vi "Avocent_Device_GUI.vi"() -> ()   [LabVIEW 2013]
doc: "Example of using standard HTTP protocol for recieving a web site (the HTML source)\n\n\nThis example uses the GET command. For general information about the HTTP protocol and other commands go to\nhttp://www.w3.org/Protocols\n\n\nBjornar Svingen\nbjornar.svingen@sintef.no bjornar.svingen@ktv.no"
uses:
  shared programs/GUI_Template/GUI_master/tcp_new_data_event.ctl
  shared programs/GUI_Template/GUI_master/tcp new data cluster.ctl
  <vilib>/Utility/config.llb/Read Key (String).vi
  <vilib>/Utility/config.llb/NI_LVConfig.lvlib
panel:
  in  "timeout::1":i32=6000 caption="timeout ms" min=0 max=0
  in  "turn selected OFF":bool
  in  "turn selected ON":bool
  out "Avocent Labels Av1":string[](array[string])
  in  "Set switches":bool[](array[boolean])=[FALSE, FALSE, FALSE, FALSE, FALSE, FALSE, FALSE, FALSE, FALSE, FALSE, FALSE, FALSE, FALSE, FALSE, FALSE, FALSE] caption="Set Switches"
  in  "Avocent IP::1":string caption="Avocent  IP"
  out "port: P::1":bool caption="port: P"
  out "port: O::1":bool caption="port: O"
  out "port: N::1":bool caption="port: N"
  out "port: M::1":bool caption="port: M"
  out "port: L::1":bool caption="port: L"
  out "port: K::1":bool caption="port: K"
  out "port: J::1":bool caption="port: J"
  out "port: I::1":bool caption="port: I"
  out "port: H::1":bool caption="port: H"
  out "port: G::1":bool caption="port: G"
  out "port: F::1":bool caption="port: F"
  out "port: E::1":bool caption="port: E"
  out "port: D::1":bool caption="port: D"
  out "port: C::1":bool caption="port: C"
  out "port: B::1":bool caption="port: B"
  out "port: A::1":bool caption="port: A"
  out "tcp data event 2":T1
  out "GUIdevice 1":string="Avocent-PSU-downstream"
  in  "Set to all on/off av1":bool
  in  "toggle av1":bool
  in  "Set to current values":bool
  out "Power indicator":bool[](array[boolean])=[FALSE, TRUE, TRUE, FALSE, TRUE, TRUE, TRUE, TRUE, TRUE, TRUE, TRUE, FALSE, TRUE, TRUE, TRUE, FALSE, FALSE, FALSE, FALSE, FALSE, FALSE, FALSE, FALSE, FALSE, FALSE, FALSE, FALSE, FALSE, FALSE, FALSE, FALSE, FALSE]
  in  "Get status":bool
  in  "send command":bool
  in  "Exit":bool
  out "Error":T2
  # "Power indicator"
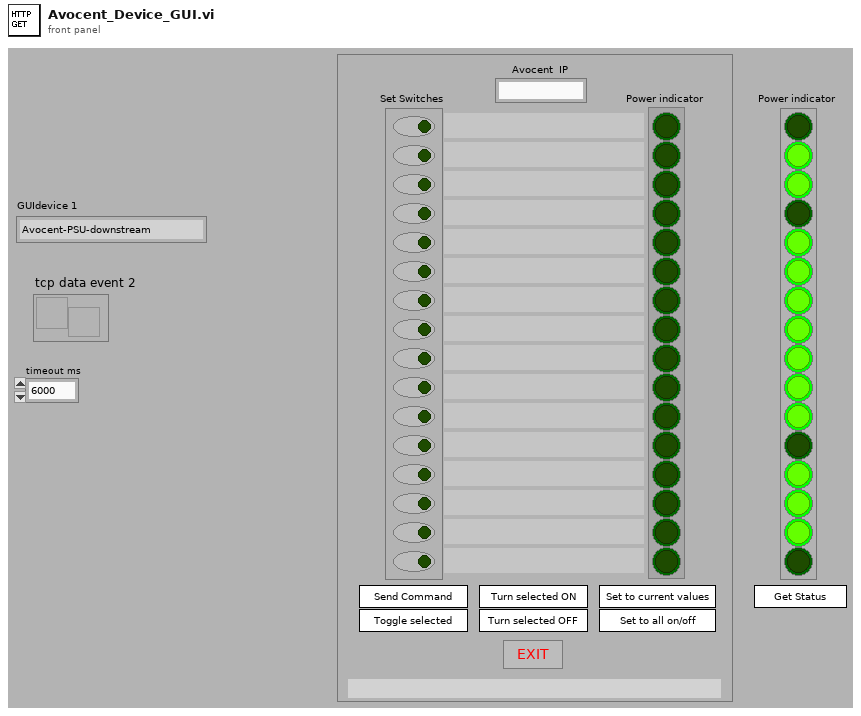
[diagram p1: front panel]
types:
  T1 = typedef "tcp_new_data_event.ctl" = refnum<user-event>
  T2 = cluster{"status":bool, "code":i32, "UDP error message":string}
  T3 = enum32{"invalid app kind", "Development System", "Run Time System", "Student Edition", "Embedded LabVIEW", "Evaluation", "Custom"}
  T4 = typedef "tcp new data cluster.ctl" = cluster{"EventEnum":enum16{"new data", "connection status update"}, "Device name":string}
  T5 = enum32{"Invalid", "Standard", "Closed", "Hidden", "Minimized", "Maximized"}
  T6 = cluster{"Core":cluster{"Current VI Reference":refnum<vi>, "Close Panel on Exit?":bool}, "HTTP Command":string, "Set Switch Status":bool[], "Power Status":string, "Toggle On/Off":bool, "Set all On/Off":bool, "SuperGUI":cluster{"STOP queue":refnum<queue>, "SuperGUI ref":refnum<vi>, "event reg":refnum<event-registration>}, "Stage Device list":string[], "Avocent IP":string}
  T7 = cluster{"STOP queue":refnum<queue>, "SuperGUI ref":refnum<vi>, "event reg":refnum<event-registration>}
  T8 = cluster{"Current VI Reference":refnum<vi>, "Close Panel on Exit?":bool}
  T9 = typedef "NI_LVConfig.lvlib/Config Data RefNum.ctl" = refnum<k1>
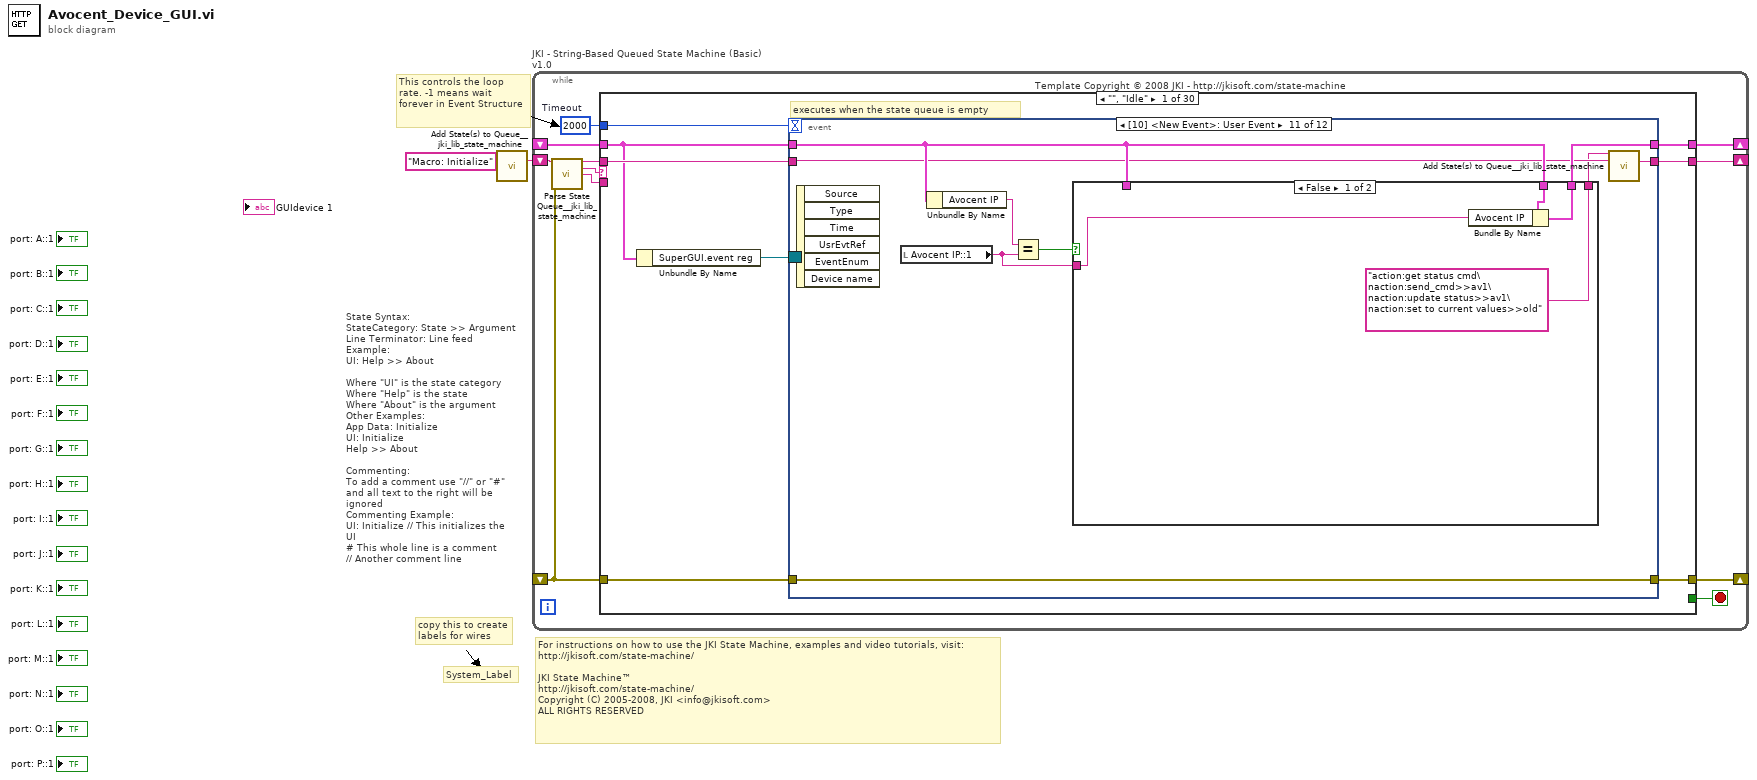
[diagram p0: block diagram]
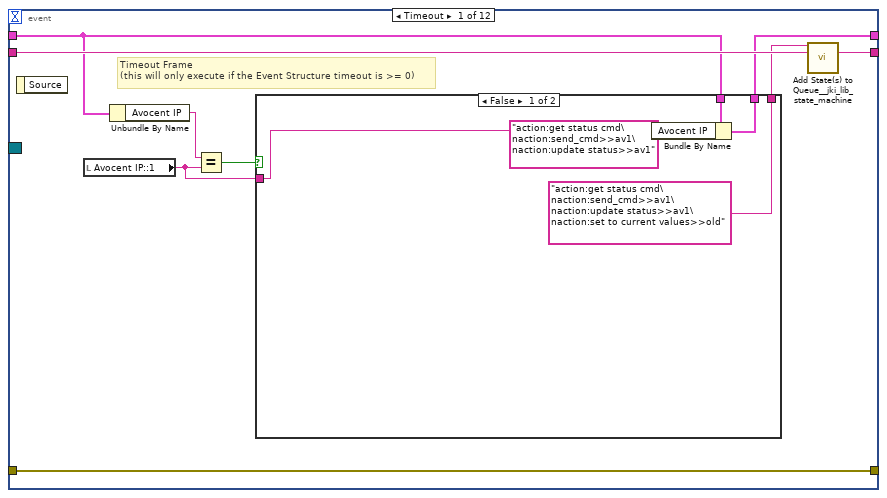
[diagram p2: hidden frame]
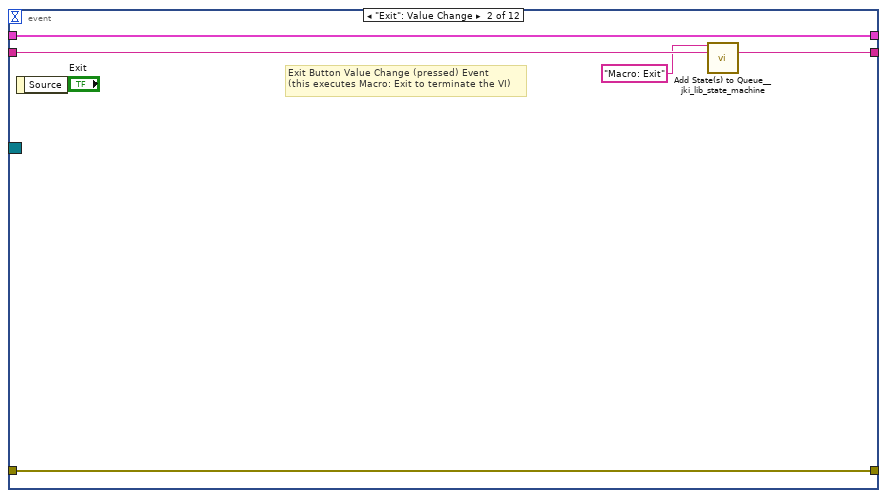
[diagram p4: hidden frame]
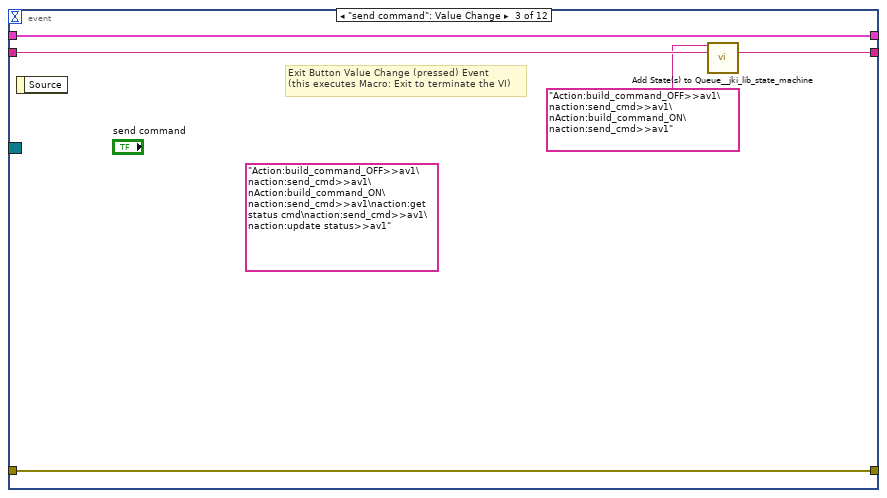
[diagram p5: hidden frame]
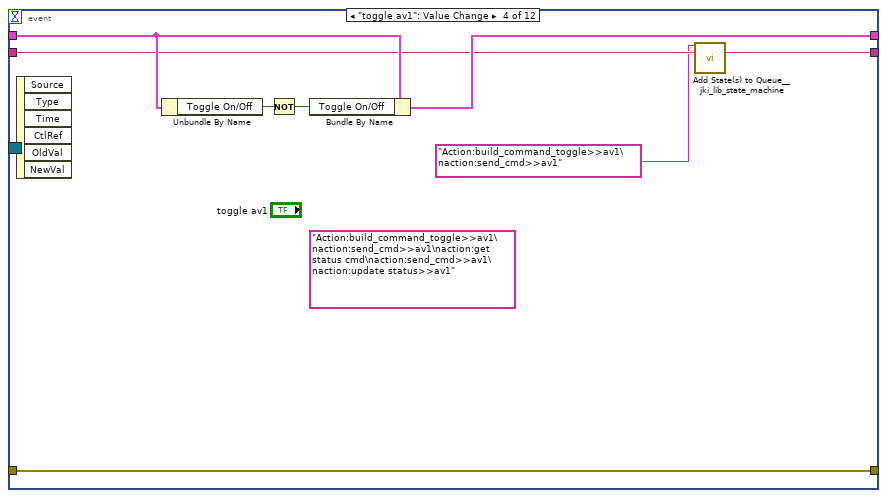
[diagram p6: hidden frame]
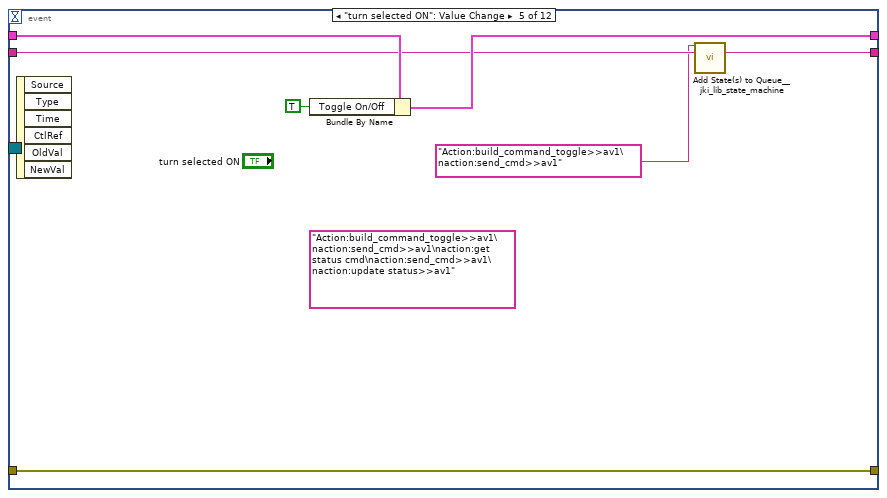
[diagram p7: hidden frame]
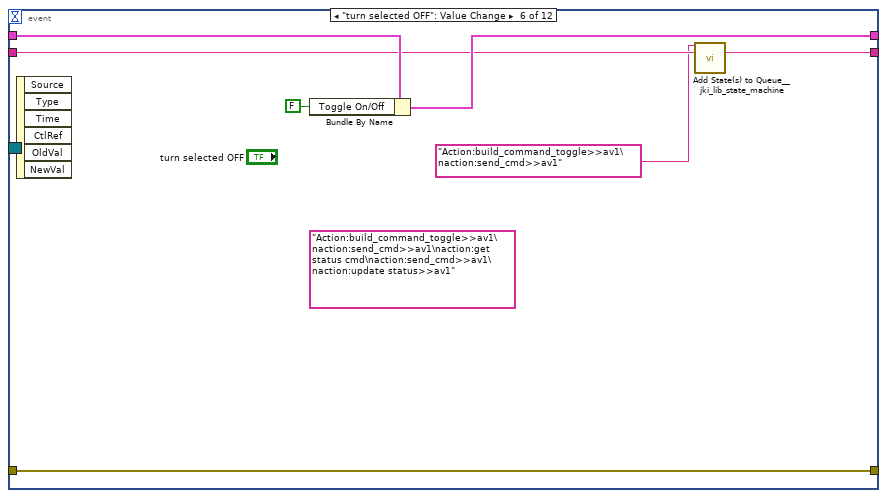
[diagram p8: hidden frame]
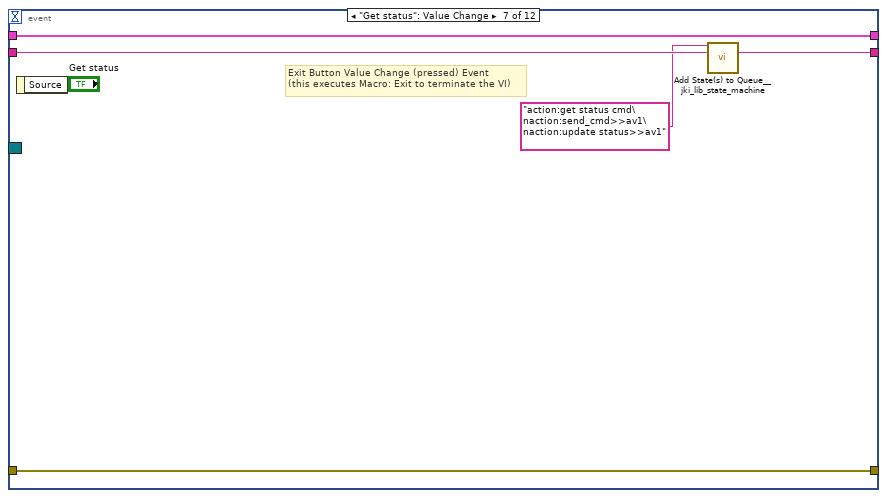
[diagram p9: hidden frame]
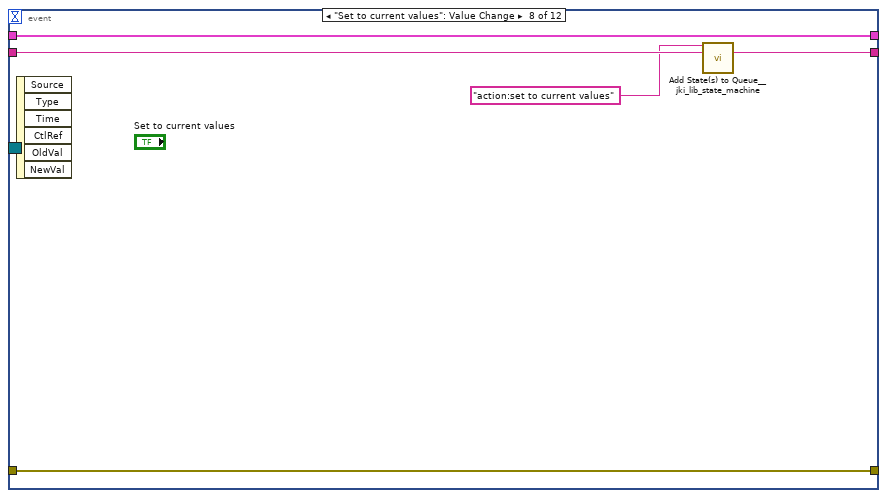
[diagram p10: hidden frame]
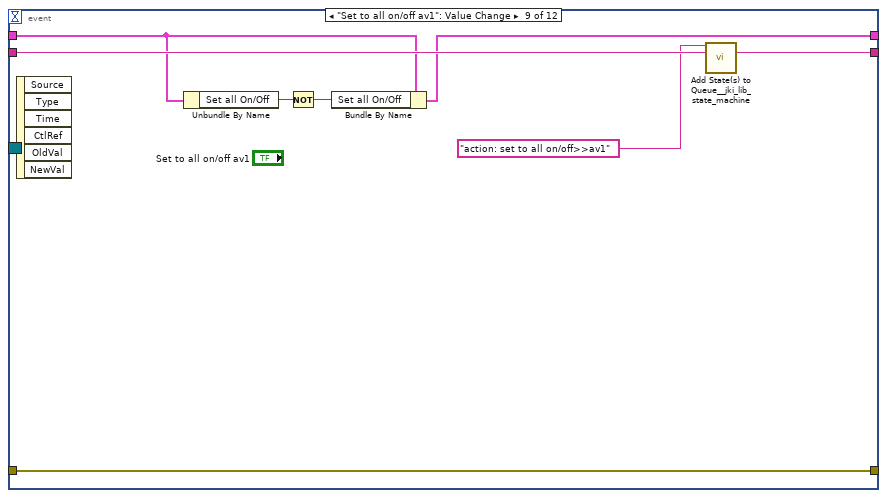
[diagram p11: hidden frame]
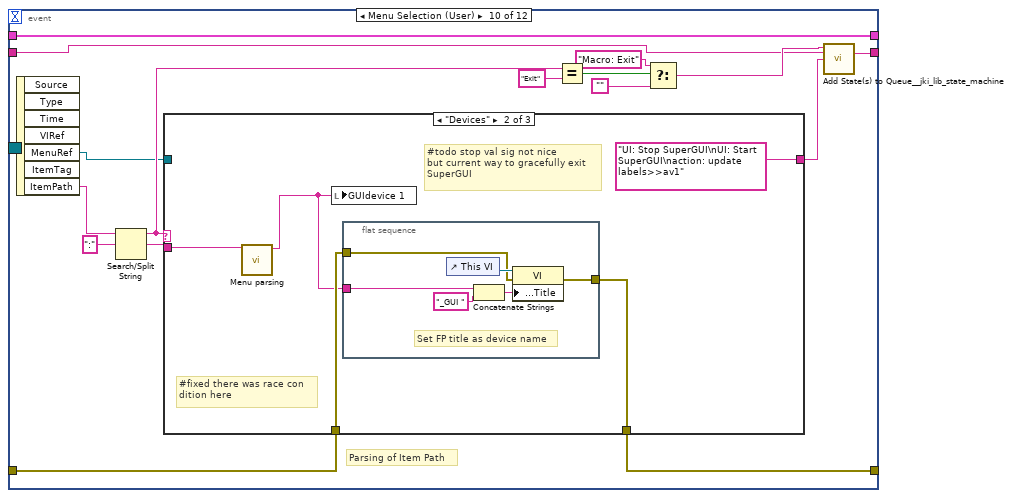
[diagram p12: hidden frame]
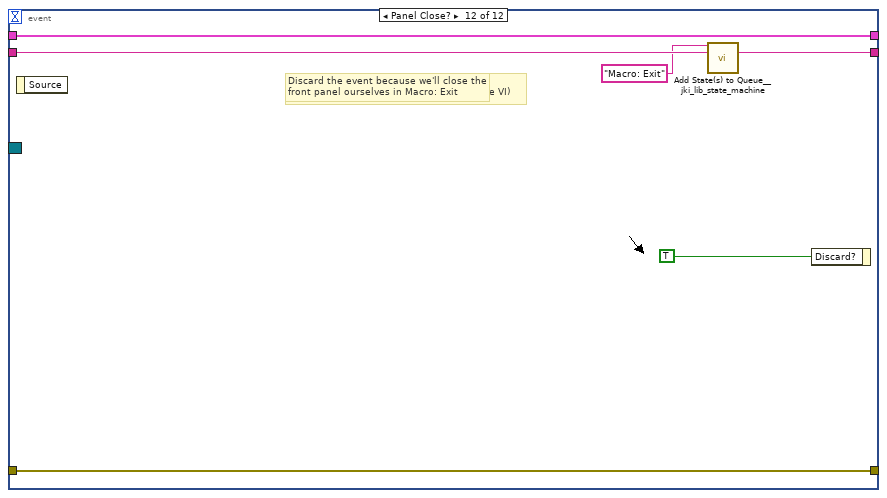
[diagram p16: hidden frame]
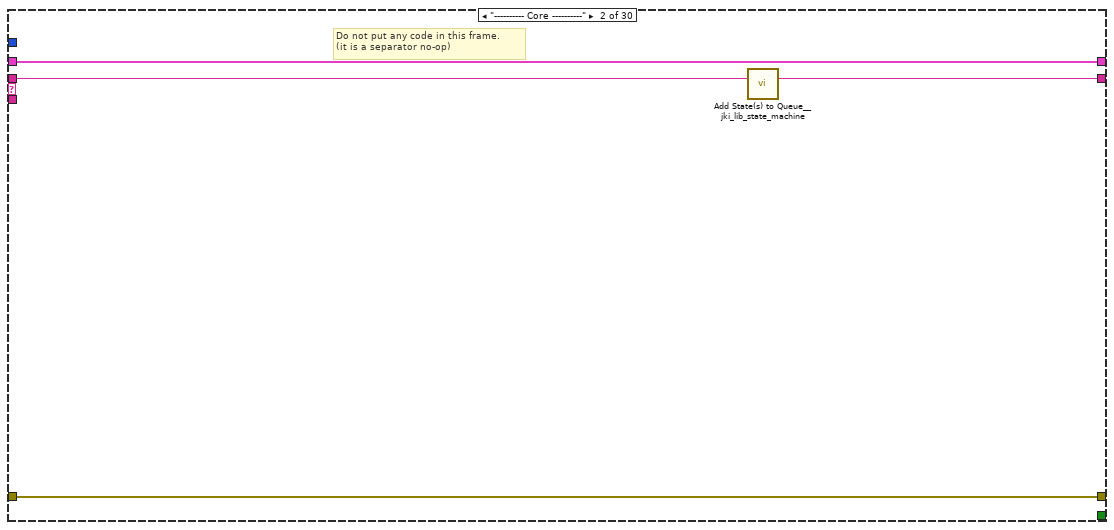
[diagram p17: hidden frame]
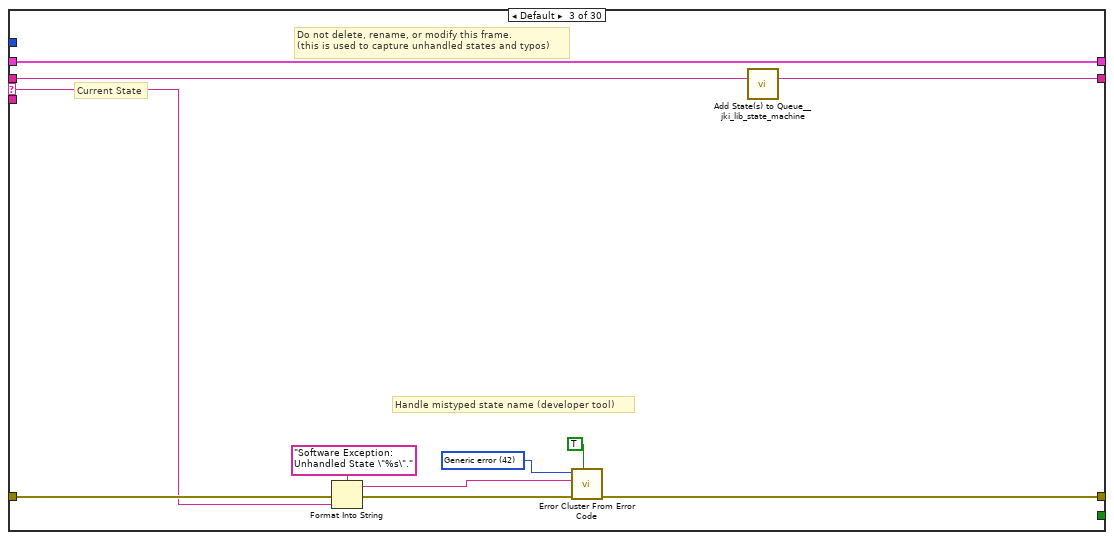
[diagram p18: hidden frame]
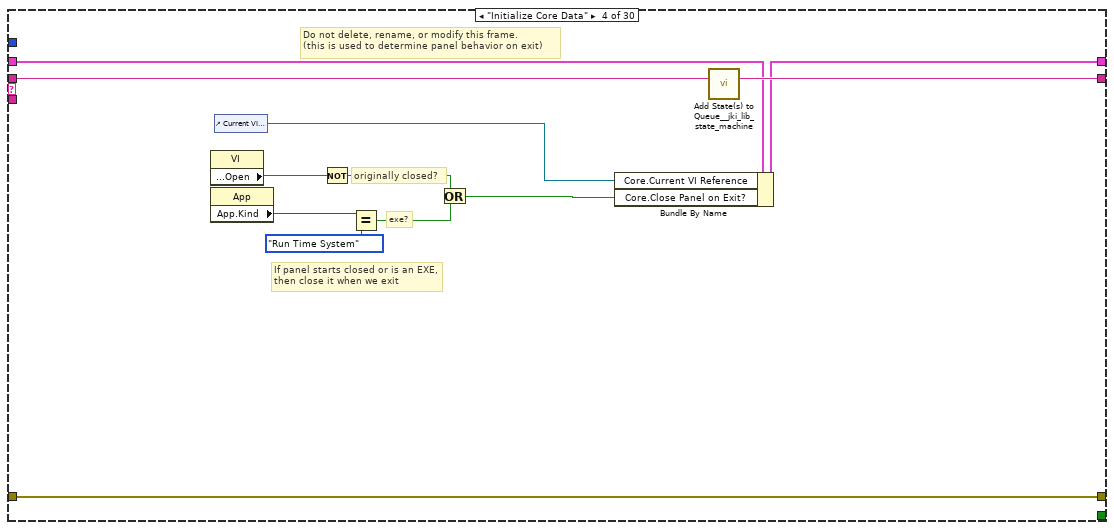
[diagram p19: hidden frame]
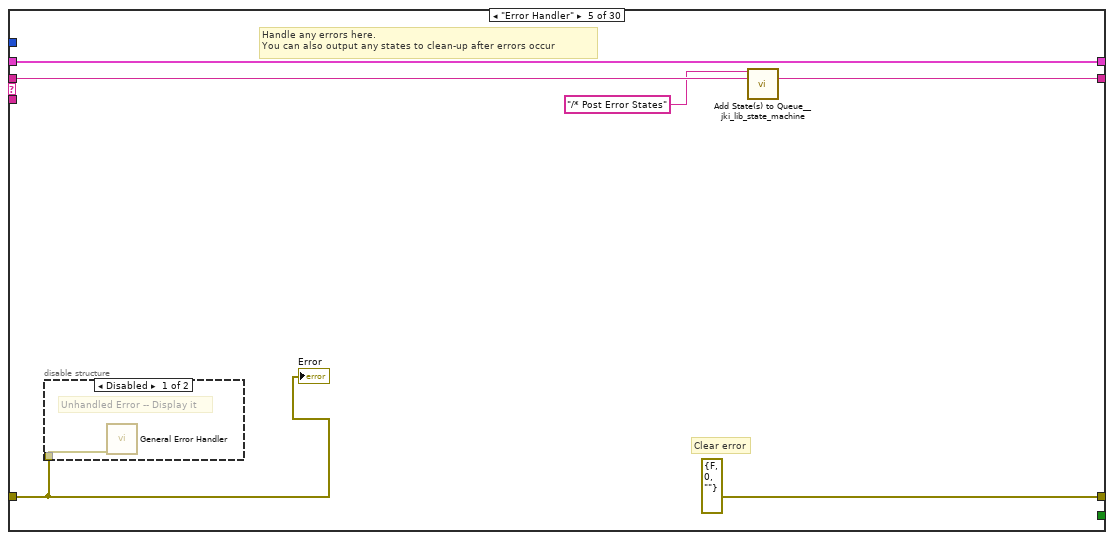
[diagram p20: hidden frame]
diagram:
  # "For instructions on how to use the JKI State Machine, examples and video tutorials, visit:\nhttp://jkisoft.com/state-machine/\n\nJKI State Machine™\nhttp://jkisoft.com/state-machine/\nCopyright (C) 2005-2008, JKI <info@jkisoft.com>\nALL RIGHTS RESERVED"
  # "State Syntax:\nStateCategory: State >> Argument\nLine Terminator: Line feed\nExample:\nUI: Help >> About\n\nWhere \"UI\" is the state category\nWhere \"Help\" is the state\nWhere \"About\" is the argument\nOther Examples:\nApp Data: Initialize\nUI: Initialize\nHelp >> About\n\nCommenting:\nTo add a comment use \"//\" or \"#\" and all text to the right will be ignored\nCommenting Example:\nUI: Initialize // This initializes the UI\n# This whole line is a comment\n// Another comment line"
  # "copy this to create labels for wires"
  # "This controls the loop rate. -1 means wait forever in Event Structure"
  # "System_Label"
  n1 = call <vilib>:"Add State(s) to Queue__jki_lib_state_machine.vi"("State(s) in (\"\")"="Macro: Initialize") -> ("States Out"=w2:string)  [unwired: 14 in]
  n2 = while "JKI - String-Based Queued State Machine (Basic) v1.0" {
    shift-right: [w6] -> _
    shift-left: _ -> [w5]
    shift-right: [w9] -> _
    shift-left: _ -> [w3]
    shift-right: [w8] -> _
    shift-left: w2 -> [w10]
    stop <- w7 stop-if-true
    w4 = 2000  # Timeout
    # "Template Copyright © 2008 JKI - http://jkisoft.com/state-machine"
    n3 = call <vilib>:"Parse State Queue__jki_lib_state_machine.vi"("State Queue"=w10, "Error In (no error)"=w3) -> ("Remaining States"=w12:string, "Current State"=w13:string, "Arguments"=w11:string)  [unwired: 11 in]
    n4 = case shown="\"\", \"Idle\"" w13 {
      selector: w13 -> [_ _ w139 _ _ _ _ _ _ _ _ _ _ _ _ _ _ _ _ _ _ _ _ _ _ _ _ _ _ _]
      tunnel: w12 -> [w21 w138 w143 w161 w167 w173 w177 w190 w196 w200 w208 w210 w231 w270 w282 w295 w306 w332 w337 w347 w351 w354 w375 w392 w397 w413 w429 w435 w463 w488]
      tunnel: w11 -> [_ _ _ _ _ _ _ _ _ _ _ _ _ _ _ w290 w300 _ _ _ _ w357 w376 _ w399 w416 _ w430 w464 w477]
      tunnel: w5 -> [w15 w135 w141 w152 w164 w171 w174 _ w191 w197 w206 w209 w232 w267 w286 w293 w302 w329 w334 w344 w348 w359 w379 w388 w398 w417 w426 w433 w459 w489]
      tunnel: [w19 w136 w145 w158 errorcluster {"status"=FALSE, "code"=0, "source"=""} ("error out") w170 w175 w187 w192 w198 w204 w212 w233 w266 w284 w291 w303 w330 w335 w345 w349 w362 w373 w390 w400 w414 w427 w431 w465 w480] -> w9
      tunnel: w3 -> [w18 w136 w144 w158 w162 w170 w175 w187 w193 w198 w205 w213 w234 w265 w285 w292 w304 w330 w335 w345 w349 w356 w374 w390 w401 w415 w427 w432 w466 w476]
      tunnel: [w20 w137 w142 w160 w166 w172 w176 w189 w195 w199 w207 w211 w231 w269 w283 w294 w305 w331 w336 w346 w350 w364 w380 w391 w403 w418 w428 w434 w467 w488] -> w8
      tunnel: [_ _ _ _ _ TRUE _ _ _ _ _ _ _ _ _ _ _ _ _ _ _ _ _ _ _ _ _ _ _ _] -> w7
      tunnel: [w17 w135 w141 w159 w164 w171 w174 w188 w191 w197 w206 w209 w232 w268 w286 w293 w302 w329 w334 w344 w348 w358 w377 w389 w402 w417 w425 w433 w459 w489] -> w6
      tunnel: w4 -> [w16 _ _ _ _ _ _ _ _ _ _ _ _ _ _ _ _ _ _ _ _ _ _ _ _ _ _ _ _ _]
      frame "", "Idle" {
        # "executes when the state queue is empty"
        n5 = Unbundle By Name(w15) -> ("SuperGUI.event reg"=w14:refnum<event-registration>)
        n6 = event shown="[10] <New Event>: User Event" {
          selector: w14 -> [_ _ _ _ _ _ _ _ _ _ _ _]
          dyn-events: _ -> [_ _ _ _ _ _ _ _ _ _ _ _]
          timeout: w16 -> [_ _ _ _ _ _ _ _ _ _ _ _]
          tunnel: w21 -> [w30 w40 w45 w48 w57 w64 w72 w74 w83 w89 w116 w134]
          tunnel: [w29 w39 w44 w47 w56 w63 w71 w75 w84 w87 w117 w133] -> w20
          tunnel: w15 -> [w23 w37 w42 w51 w58 w65 w69 w77 w79 w88 w119 w131]
          tunnel: [w28 w38 w43 w53 w60 w67 w70 w76 w85 w93 w123 w132] -> w19
          tunnel: w18 -> [w28 w38 w43 w53 w60 w67 w70 w76 w85 w92 w123 w132]
          tunnel: [w22 w37 w42 w52 w59 w66 w69 w77 w78 w88 w121 w131] -> w17
          event Timeout {
            (unwired) "action:get status cmd\naction:send_cmd>>av1\naction:update status>>av1"
            # "Timeout Frame\n(this will only execute if the Event Structure timeout is >= 0)"
            n7 = event-data() -> ()  [unwired: 1 in, 1 out]
            n8 = local read "Avocent IP::1"() -> (w25:string)
            n9 = Unbundle By Name(w23) -> ("Avocent IP"=w27:string)
            n10 = Equal?(x=w27, y=w25) -> (x = y?=w26:bool)
            n11 = case shown="False" w26 {
              tunnel: w23 -> [w34 w35]
              tunnel: [w33 w35] -> w22
              tunnel: w25 -> [w32 _]
              tunnel: ["action:get status cmd\naction:send_cmd>>av1\naction:update status>>av1\naction:set to current values>>old" ("State(s) in Front (\"\")") _] -> w24
              frame False {
                n12 = Bundle By Name(cluster=w34, "Avocent IP"=w32) -> (w33:T6)
              }
              frame True {
              }
            }
            n13 = call <vilib>:"Add State(s) to Queue__jki_lib_state_machine.vi"("State(s) in Front (\"\")"=w24, "State(s) in (\"\")"=w30) -> ("States Out"=w29:string)  [unwired: 13 in]
          }
          event "Exit": Value Change {
            # "Exit Button Value Change (pressed) Event\n(this executes Macro: Exit to terminate the VI)"
            n14 = event-data() -> ()  [unwired: 1 in, 1 out]
            n15 = call <vilib>:"Add State(s) to Queue__jki_lib_state_machine.vi"("State(s) in Front (\"\")"="Macro: Exit", "State(s) in (\"\")"=w40) -> ("States Out"=w39:string)  [unwired: 13 in]
          }
          event "send command": Value Change {
            (unwired) "Action:build_command_OFF>>av1\naction:send_cmd>>av1\nAction:build_command_ON\naction:send_cmd>>av1\naction:get status cmd\naction:send_cmd>>av1\naction:update status>>av1"
            # "Exit Button Value Change (pressed) Event\n(this executes Macro: Exit to terminate the VI)"
            n16 = event-data() -> ()  [unwired: 1 in, 1 out]
            n17 = call <vilib>:"Add State(s) to Queue__jki_lib_state_machine.vi"("State(s) in Front (\"\")"="Action:build_command_OFF>>av1\naction:send_cmd>>av1\nAction:build_command_ON\naction:send_cmd>>av1", "State(s) in (\"\")"=w45) -> ("States Out"=w44:string)  [unwired: 13 in]
          }
          event "toggle av1": Value Change {
            (unwired) "Action:build_command_toggle>>av1\naction:send_cmd>>av1\naction:get status cmd\naction:send_cmd>>av1\naction:update status>>av1"
            n18 = event-data() -> ()  [unwired: 1 in, 6 out]
            n19 = Unbundle By Name(w51) -> ("Toggle On/Off"=w50:bool)
            n20 = Not(x=w50) -> (.not. x?=w49:bool)
            n21 = Bundle By Name(cluster=w51, "Toggle On/Off"=w49) -> (w52:T6)
            n22 = call <vilib>:"Add State(s) to Queue__jki_lib_state_machine.vi"("State(s) in Front (\"\")"="Action:build_command_toggle>>av1\naction:send_cmd>>av1", "State(s) in (\"\")"=w48) -> ("States Out"=w47:string)  [unwired: 13 in]
          }
          event "turn selected ON": Value Change {
            (unwired) "Action:build_command_toggle>>av1\naction:send_cmd>>av1\naction:get status cmd\naction:send_cmd>>av1\naction:update status>>av1"
            n23 = event-data() -> ()  [unwired: 1 in, 6 out]
            n24 = Bundle By Name(cluster=w58, "Toggle On/Off"=TRUE) -> (w59:T6)
            n25 = call <vilib>:"Add State(s) to Queue__jki_lib_state_machine.vi"("State(s) in Front (\"\")"="Action:build_command_toggle>>av1\naction:send_cmd>>av1", "State(s) in (\"\")"=w57) -> ("States Out"=w56:string)  [unwired: 13 in]
          }
          event "turn selected OFF": Value Change {
            (unwired) "Action:build_command_toggle>>av1\naction:send_cmd>>av1\naction:get status cmd\naction:send_cmd>>av1\naction:update status>>av1"
            n26 = event-data() -> ()  [unwired: 1 in, 6 out]
            n27 = Bundle By Name(cluster=w65, "Toggle On/Off"=FALSE) -> (w66:T6)
            n28 = call <vilib>:"Add State(s) to Queue__jki_lib_state_machine.vi"("State(s) in Front (\"\")"="Action:build_command_toggle>>av1\naction:send_cmd>>av1", "State(s) in (\"\")"=w64) -> ("States Out"=w63:string)  [unwired: 13 in]
          }
          event "Get status": Value Change {
            # "Exit Button Value Change (pressed) Event\n(this executes Macro: Exit to terminate the VI)"
            n29 = event-data() -> ()  [unwired: 1 in, 1 out]
            n30 = call <vilib>:"Add State(s) to Queue__jki_lib_state_machine.vi"("State(s) in Front (\"\")"="action:get status cmd\naction:send_cmd>>av1\naction:update status>>av1", "State(s) in (\"\")"=w72) -> ("States Out"=w71:string)  [unwired: 13 in]
          }
          event "Set to current values": Value Change {
            n31 = event-data() -> ()  [unwired: 1 in, 6 out]
            n32 = call <vilib>:"Add State(s) to Queue__jki_lib_state_machine.vi"("State(s) in Front (\"\")"="action:set to current values" ("State(s) in Front (\"\")"), "State(s) in (\"\")"=w74) -> ("States Out"=w75:string)  [unwired: 13 in]
          }
          event "Set to all on/off av1": Value Change {
            n33 = event-data() -> ()  [unwired: 1 in, 6 out]
            n34 = Unbundle By Name(w79) -> ("Set all On/Off"=w81:bool)
            n35 = Not(x=w81) -> (.not. x?=w80:bool)
            n36 = Bundle By Name(cluster=w79, "Set all On/Off"=w80) -> (w78:T6)
            n37 = call <vilib>:"Add State(s) to Queue__jki_lib_state_machine.vi"("State(s) in Front (\"\")"="action: set to all on/off>>av1" ("State(s) in Front (\"\")"), "State(s) in (\"\")"=w83) -> ("States Out"=w84:string)  [unwired: 13 in]
          }
          event Menu Selection (User) {
            # "Parsing of Item Path"
            n38 = event-data() -> ("MenuRef"=w91:refnum<k9>, "ItemPath"=w90:string)  [unwired: 1 in, 5 out]
            n39 = Search/Split String(string=w90, search string/char (-)=":") -> (substring before match=w100:string, match + rest of string=w94:string)  [unwired: 1 in, 1 out]
            n40 = case shown="\"Devices\"" w100 {
              tunnel: w94 -> [_ w107 _]
              tunnel: w91 -> [_ _ _]
              tunnel: w92 -> [w102 w106 w114]
              tunnel: [w102 w105 w114] -> w93
              tunnel: [_ "UI: Stop SuperGUI\nUI: Start SuperGUI\naction: update labels>>av1" _] -> w101
              frame "", Default {
              }
              frame "Devices" {
                # "#fixed there was race con\ndition here"
                # "#todo stop val sig not nice\nbut current way to gracefully exit\nSuperGUI"
                n41 = call "Menu parsing.vi"("ItemPath 3"=w107) -> ("ItemPath 2"=w103:string)  [unwired: 9 in, 1 out]
                n42 = local write "GUIdevice 1"(w103) -> ()
                n43 = flat-sequence {
                  tunnel: [w110] -> w105
                  tunnel: w106 -> [w109]
                  tunnel: w103 -> [w108]
                  frame #0 {
                    # "Set FP title as device name"
                    n44 = control-ref of="This VI"() -> (w113:refnum<vi>)
                    n45 = Concatenate Strings(w108, "_GUI ") -> (w112:string)
                    n46 = property class="VI"(reference=w113, error in=w109, "Front Panel.Title"=w112) -> (error out=w110:errorcluster)  [unwired: 1 out]
                  }
                }
              }
              frame "Exit" {
              }
            }
            n47 = Equal?(x=w100, y="Exit") -> (x = y?=w96:bool)
            n48 = Select(t="Macro: Exit", s=w96, f="") -> (s? t:f=w99:string)
            n49 = call <vilib>:"Add State(s) to Queue__jki_lib_state_machine.vi"("State(s) in Front (\"\")"=w99, "State(s) in (\"\")"=w89, "State(s) at Back (\"\")"=w101) -> ("States Out"=w87:string)  [unwired: 12 in]
          }
          event User Event {
            n50 = event-data() -> ()  [unwired: 1 in, 6 out]
            n51 = local read "Avocent IP::1"() -> (w118:string)
            n52 = Unbundle By Name(w119) -> ("Avocent IP"=w122:string)
            n53 = Equal?(x=w122, y=w118) -> (x = y?=w120:bool)
            n54 = case shown="False" w120 {
              tunnel: w119 -> [w127 w128]
              tunnel: [w126 w128] -> w121
              tunnel: w118 -> [w125 _]
              tunnel: w119 -> [_ _]
              tunnel: ["action:get status cmd\naction:send_cmd>>av1\naction:update status>>av1\naction:set to current values>>old" ("State(s) in Front (\"\")") _] -> w115
              frame False {
                n55 = Bundle By Name(cluster=w127, "Avocent IP"=w125) -> (w126:T6)
              }
              frame True {
              }
            }
            n56 = call <vilib>:"Add State(s) to Queue__jki_lib_state_machine.vi"("State(s) in Front (\"\")"=w115, "State(s) in (\"\")"=w116) -> ("States Out"=w117:string)  [unwired: 13 in]
          }
          event Panel Close? {
            # "Discard the event because we'll close the front panel ourselves in Macro: Exit"
            # "Close Panel button (pressed) Event\n(this executes Macro: Exit to terminate the VI)"
            n57 = event-data() -> ()  [unwired: 1 in, 1 out]
            n58 = call <vilib>:"Add State(s) to Queue__jki_lib_state_machine.vi"("State(s) in Front (\"\")"="Macro: Exit", "State(s) in (\"\")"=w134) -> ("States Out"=w133:string)  [unwired: 13 in]
            n59 = event-data("Discard?"=TRUE) -> ()  [unwired: 1 in, 1 out]
          }
        }
      }
      frame "---------- Core ----------" {
        # "Do not put any code in this frame.\n(it is a separator no-op)"
        n60 = call <vilib>:"Add State(s) to Queue__jki_lib_state_machine.vi"("State(s) in (\"\")"=w138) -> ("States Out"=w137:string)  [unwired: 14 in]
      }
      frame Default {
        w148 = 42 items=["No error", "Argument error", "Memory is full", "Out of zone", "End of file", "File already open", "Generic file I/O error", "File not found", "File permission error", "Disk is full", "Duplicate path", "Too many files open", "System feature not enabled", "Resource file not found", "Cannot add resource", "Resource not found", "Image not found", "Image memory error", "Pen does not exist", "Config type invalid", "Config token not found", "Config parse error", "Config memory error", "Bad external code format", "Bad external code offset", "External code not present", "Null window", "Destroy window error", "Null menu", "Print aborted", "Bad print record", "Print driver error", "Windows error during printing", "Memory error during printing", "Print dialog error", "Generic print error", "Invalid device refnum", "Device not found", "Device parameter error", "Device unit error", "Cannot open device", "Device call aborted", "Generic error", "Cancelled by user", "Object ID too low", "Object ID too high", "Object not in heap", "Unknown heap", "Unknown object (invalid DefProc)", "Unknown object (DefProc not in table)", "Message out of range", "Invalid (null) method", "Unknown message", "Manager call not supported", "Bad address", "Network operation in progress", "Network operation timed out", "Connection is busy", "Network attribute not supported", "Network error", "Address in use", "System out of memory", "Connection aborted", "Connection refused", "Not connected", "Already connected", "Connection closed", "Initialization error (interapplication manager)", "Bad occurrence", "Wait on unbound occurrence handler", "Occurrence queue overflow", "Datalog type conflict", "Unused", "Unrecognized type (interapplication manager)", "Memory corrupt", "Failed to make temporary DLL", "Old CIN version", "Drag socket not found", "Failed to load drop-object", "Failed to register OLE object", "Failed to release OLE object", "Format specifier type mismatch", "Unknown format specifier", "Too few format specifiers", "Too many format specifiers", "Scan failed", "Newer CIN version", "Error converting to variant", "Runtime menu error", "Password tampered", "Variant attribute not found", "Incompatible variant data type", "Event data is not available", "Event Store is not present", "Occurrence is not found", "Event Queue is not created", "Event info is not available", "Refnum passed is NULL", "Error retrieving Class GUID", "Error retrieving CoClass GUID", "Error retrieving TypeLib GUID.", "Bad built application magic bytes.", "Specific driver is different from the specific driver associated with the Logical Name.", "There is no session opened to the class driver.", "Max Error", "MAX - Error with config objects", "MAX - Error loading configuration", "MAX - Group not supported"]
        # "Current State"
        # "Do not delete, rename, or modify this frame.\n(this is used to capture unhandled states and typos)"
        # "Handle mistyped state name (developer tool)"
        n61 = Format Into String(format string="Software Exception: Unhandled State \"%s\"." ("message"), error in=w144, w139) -> (resulting string=w147:string, error out=w146:errorcluster)  [unwired: 1 in]
        n62 = call <vilib>:"Error Cluster From Error Code.vi"("show call chain? (False)"=TRUE, "error in (no error)"=w146, "error message (\"\")"=w147, "error code (0)"=w148) -> ("error out"=w145:errorcluster)  [unwired: 5 in]
        n63 = call <vilib>:"Add State(s) to Queue__jki_lib_state_machine.vi"("State(s) in (\"\")"=w143) -> ("States Out"=w142:string)  [unwired: 14 in]
      }
      frame "Initialize Core Data" {
        # "Do not delete, rename, or modify this frame.\n(this is used to determine panel behavior on exit)"
        # "originally closed?"
        # "exe?"
        # "If panel starts closed or is an EXE, then close it when we exit"
        n64 = property class="VI"() -> ("Front Panel.Open"=w157:bool)  [unwired: 2 in, 2 out]
        n65 = property class="App"() -> ("App.Kind"=w156:T3)  [unwired: 2 in, 2 out]
        n66 = control-ref of="Current VI Reference"() -> (w150:refnum<vi>)
        n67 = Not(x=w157) -> (.not. x?=w154:bool)
        n68 = Equal?(x=w156, y=T3."Run Time System" ("Application:Kind")) -> (x = y?=w153:bool)
        n69 = Or(x=w154, y=w153) -> (x .or. y?=w151:bool)
        n70 = Bundle By Name(cluster=w152, "Core.Current VI Reference"=w150, "Core.Close Panel on Exit?"=w151) -> (w159:T6)
        n71 = call <vilib>:"Add State(s) to Queue__jki_lib_state_machine.vi"("State(s) in (\"\")"=w161) -> ("States Out"=w160:string)  [unwired: 14 in]
      }
      frame "Error Handler" {
        # "Handle any errors here.\nYou can also output any states to clean-up after errors occur"
        # "Clear error"
        n72 = disable-structure shown="Disabled" {
          disable-tunnel: w162 -> [w168 _]
          frame Disabled {
            # "Unhandled Error -- Display it"
            n73 = call <vilib>:"General Error Handler.vi"("error in (no error)"=w168) -> ()  [unwired: 10 in, 5 out]
          }
          frame Enabled {
          }
        }
        n74 = call <vilib>:"Add State(s) to Queue__jki_lib_state_machine.vi"("State(s) in Front (\"\")"="/* Post Error States", "State(s) in (\"\")"=w167) -> ("States Out"=w166:string)  [unwired: 13 in]
        "Error" <- w162
      }
      frame "Exit" {
        # "Do not put any code in this frame.\n(No errors that occur here will be handled.)"
        n75 = call <vilib>:"Add State(s) to Queue__jki_lib_state_machine.vi"("State(s) in (\"\")"=w173) -> ("States Out"=w172:string)  [unwired: 14 in]
      }
      frame "---------- Data ----------" {
        # "Do not put any code in this frame.\n(It is a separator no-op. You can make a copy of this frame to create a new Data frame)"
        n76 = call <vilib>:"Add State(s) to Queue__jki_lib_state_machine.vi"("State(s) in (\"\")"=w177) -> ("States Out"=w176:string)  [unwired: 14 in]
      }
      frame "Data: Initialize" {
        w178 = ""  # Avocent IP
        w179 = string[] []  # Stage Device list
        w180 = T7 {"STOP queue"=refnum, "SuperGUI ref"=refnum, "event reg"=refnum}  # SuperGUI
        w181 = TRUE  # Set all On/Off
        w182 = bool[] [FALSE, FALSE, FALSE, FALSE, FALSE, FALSE, FALSE, FALSE, FALSE, TRUE, FALSE, FALSE, FALSE, FALSE, FALSE, FALSE, FALSE, FALSE, FALSE, FALSE, FALSE, FALSE, FALSE, FALSE, FALSE, FALSE, FALSE, FALSE, FALSE, FALSE, FALSE, FALSE]  # Set Switch Status
        w183 = TRUE  # Toggle On/Off
        w184 = ""  # Power Status
        w185 = ""  # HTTP Command
        w186 = T8 {"Current VI Reference"=refnum, "Close Panel on Exit?"=FALSE}  # Core
        # "do not delete - used by framework"
        # "Data names and types of shift register data are defined by this bundle."
        # "Initialize the shift-register data, here.\n(data names are defined by what you wire into the bundle function)"
        n77 = Bundle("Core"=w186, "HTTP Command"=w185, "Set Switch Status"=w182, "Power Status"=w184, "Toggle On/Off"=w183, "Set all On/Off"=w181, "SuperGUI"=w180, "Stage Device list"=w179, "Avocent IP"=w178) -> (w188:T6)  [unwired: 1 in]
        n78 = call <vilib>:"Add State(s) to Queue__jki_lib_state_machine.vi"("State(s) in (\"\")"=w190) -> ("States Out"=w189:string)  [unwired: 14 in]
      }
      frame "Data: Cleanup" {
        # "Cleanup any data and references, here.\n(this is called automatically, by the Macro: Exit)"
        n79 = Unbundle By Name(w191) -> ("Core.Current VI Reference"=w194:refnum<vi>)
        n80 = Close Reference(reference=w194, error in (no error)=w193) -> (error out=w192:errorcluster)
        n81 = call <vilib>:"Add State(s) to Queue__jki_lib_state_machine.vi"("State(s) in (\"\")"=w196) -> ("States Out"=w195:string)  [unwired: 14 in]
      }
      frame "---------- UI ----------" {
        # "Do not put any code in this frame.\n(It is a separator no-op. You can make a copy of this frame to create a new UI frame)"
        n82 = call <vilib>:"Add State(s) to Queue__jki_lib_state_machine.vi"("State(s) in (\"\")"=w200) -> ("States Out"=w199:string)  [unwired: 14 in]
      }
      frame "UI: Initialize" {
        # "Edit mode untill Device list doesnt \nget update in runtime menu"
        # "Initialize the User Interface, here.\n(this is called automatically, by the Macro: Init)"
        n83 = control-ref of="This VI"() -> (w202:refnum<vi>)
        n84 = property class="VI"(reference=w202, "Edit Mode"=FALSE ("Edit Mode On Open")) -> ()  [unwired: 1 in, 2 out]
        n85 = call <userlib>:"Fit VI window to Largest Dec__ogtk.vi"("error in (no error)"=w205, "border spacing (2 px)"=-3) -> ("error out"=w204:errorcluster)  [unwired: 4 in, 1 out]
        n86 = call <vilib>:"Add State(s) to Queue__jki_lib_state_machine.vi"("State(s) in (\"\")"=w208) -> ("States Out"=w207:string)  [unwired: 14 in]
      }
      frame "UI: Get Device Name" {
        n87 = First Call?() -> (First Call?: T/F=w214:bool)
        n88 = case shown="True" w214 {
          tunnel: w213 -> [w215 w217]
          tunnel: [w215 w216] -> w212
          frame False {
          }
          frame True {
            n89 = disable-structure "Get Device name from control for vi mode\nand command line arg for exe" shown="RUN_TIME_ENGINE==True" {
              disable-tunnel: w217 -> [_ w219]
              disable-tunnel: [_ w218] -> w216
              frame condition #0 (active) {
              }
              frame condition #1 {
                n90 = control-ref of="This Application"() -> (w227:refnum<vi>)
                n91 = property class="App"(reference=w227) -> ("App.Args"=w226:string[])  [unwired: 1 in, 2 out]
                n92 = Index Array(array=w226, index #1=1 ("index")) -> (element #1=w220:string)  [unwired: 2 in, 2 out]
                n93 = Empty String/Path?(string/path=w220) -> (empty?=w224:bool)
                n94 = control-ref of="This VI"() -> (w223:refnum<vi>)
                n95 = case shown="False" w224 {
                  tunnel: w220 -> [w228 _]
                  frame False {
                    n96 = local write "GUIdevice 1"(w228) -> ()
                  }
                  frame True {
                  }
                }
                n97 = Concatenate Strings(w220, "_GUI ") -> (w222:string)
                n98 = property class="VI"(reference=w223, error in=w219, "Front Panel.Title"=w222) -> (error out=w218:errorcluster)  [unwired: 1 out]
              }
            }
          }
        }
        n99 = call <vilib>:"Add State(s) to Queue__jki_lib_state_machine.vi"("State(s) in (\"\")"=w210) -> ("States Out"=w211:string)  [unwired: 14 in]
      }
      frame "UI: Update Device List" {
        # "#todo this should be in database"
        n100 = Current VI's Menubar() -> (w244:refnum<k9>)
        n101 = Get Menu Item Info(7:"Devices" ("item tag"), 8:w234, 11:w244) -> (0:w237:errorcluster, 3:w242:refnum<k9>)  [unwired: 5 out]
        n102 = for {
          tunnel: [w248] -> w229 mode=concatenating
          tunnel: string[] ["AvocentPSU"] -> [w247] mode=indexing
          n103 = call "getDevices.vi"("Device Class"=w247) -> ("All Devices"=w248:string[])
        }
        n104 = Set Menu Item Info(7:"Devices" ("item tag"), 8:w237, 9:TRUE ("enabled"), 11:w242) -> (0:w238:errorcluster, 3:w240:refnum<k9>)  [unwired: 3 in]
        n105 = First Call?() -> (First Call?: T/F=w246:bool)
        n106 = case shown="True" w246 {
          tunnel: w240 -> [_ w254]
          tunnel: w229 -> [_ w253]
          tunnel: w238 -> [w249 w251]
          tunnel: [w249 w250] -> w236
          frame False {
          }
          frame True {
            n107 = for {
              tunnel: [w261] -> w255
              tunnel: w253 -> [w259] mode=indexing
              tunnel: w254 -> [w258]
              tunnel: [w257] -> w252
              tunnel: w251 -> [w256]
              n108 = Insert Menu Items(5:"Devices" ("menu tag"), 6:w256, 7:w259, 8:w259, 9:w258) -> (0:w257:errorcluster, 3:w261:refnum<k9>)  [unwired: 1 in, 1 out]
            }
            n109 = Enable Menu Tracking(2:w252, 4:w255) -> (0:w250:errorcluster)  [unwired: 1 in, 1 out]
          }
        }
        n110 = control-ref of="This VI"() -> (w235:refnum<vi>)
        n111 = property class="VI"(reference=w235, error in=w236, "Edit Mode"=TRUE ("Edit Mode On Open")) -> (error out=w233:errorcluster)  [unwired: 1 out]
      }
      frame "UI: Start SuperGUI" {
        # "create stop queue for supergui and its clones"
        # "x100 abort will be dependent on caller VI\nx80 abort will be independent of caller vi, this will abort vi when labview is closed."
        n112 = vi-ref "GUI_Master_subvi_reentrant_queues.vi"() -> (w273:refnum<vi>)
        n113 = Create User Event(user event datatype=T4 {"EventEnum"=enum."new data", "Device name"="Device name"} ("New Event")) -> (user event=w263:refnum<user-event>)  [unwired: 1 in, 1 out]
        "tcp data event 2" <- w263
        n114 = register-events(w263) -> (reference out=w262:refnum<event-registration>)  [unwired: 2 in, 1 out]
        n115 = property class="VI"(reference=w273) -> ("Path"=w272:path)  [unwired: 1 in, 2 out]
        n116 = control-ref of="This Application"() -> (w276:refnum<vi>)
        n117 = control-ref of="This VI"() -> (w275:refnum<vi>)
        n118 = Open VI Reference(type specifier VI Refnum (for type only)=refnum<vi> refnum, vi path=w272, options=256) -> (vi reference=w281:refnum<vi>, error out=w280:errorcluster)  [unwired: 3 in]
        n119 = call "supergui create stop queue.vi"() -> ("STOP Queue out"=w277:refnum<queue>)  [unwired: 11 in]
        n120 = Current VI's Menubar() -> (w274:refnum<k9>)
        n121 = call-by-ref "Start Asynchronous Call"(reference=w281, error in=w280, "STOP Queue in"=w277, "This Application"=w276, 8:"error in (no error)"=w265, "tcp data event"=w263, "Caller menu reference"=w274, "Caller VI ref"=w275) -> (reference out=w271:refnum<vi>, error out=w266:errorcluster)  [unwired: 5 in, 1 out]
        n122 = Bundle By Name(cluster=w267, "SuperGUI.event reg"=w262, "SuperGUI.SuperGUI ref"=w271, "SuperGUI.STOP queue"=w277) -> (w268:T6)
        n123 = call <vilib>:"Add State(s) to Queue__jki_lib_state_machine.vi"("State(s) in (\"\")"=w270) -> ("States Out"=w269:string)  [unwired: 14 in]
      }
      frame "UI: Stop SuperGUI" {
        n124 = Unbundle By Name(w286) -> ("SuperGUI.SuperGUI ref"=w288:refnum<vi>, "SuperGUI.STOP queue"=w287:refnum<queue>)
        n125 = Release Queue(queue=w287, error in (no error)=w285) -> (error out=w289:errorcluster)  [unwired: 1 in, 2 out]
        n126 = call-by-ref "Wait On Asynchronous Call"(reference=w288, error in=w289) -> ("error out"=w284:errorcluster)  [unwired: 11 in, 2 out]
        n127 = call <vilib>:"Add State(s) to Queue__jki_lib_state_machine.vi"("State(s) in (\"\")"=w282) -> ("States Out"=w283:string)  [unwired: 14 in]
      }
      frame "UI: Cursor Set" {
        # "Argument"
        # "Set and Unset Cursor Busy.\n(Usage: \"UI: Cursor Set >> Busy|Idle\")"
        n128 = case shown="\"Idle\", Default" w290 {
          tunnel: w292 -> [w297 w299]
          tunnel: [w296 w298] -> w291
          frame "Idle", Default {
            n129 = call <vilib>:"Unset Busy.vi"("error in (no error)"=w297) -> ("error out"=w296:errorcluster)  [unwired: 10 in]
          }
          frame "Busy" {
            n130 = call <vilib>:"Set Busy.vi"("error in (no error)"=w299) -> ("error out"=w298:errorcluster)  [unwired: 9 in, 1 out]
          }
        }
        n131 = call <vilib>:"Add State(s) to Queue__jki_lib_state_machine.vi"("State(s) in (\"\")"=w295) -> ("States Out"=w294:string)  [unwired: 14 in]
      }
      frame "UI: Front Panel State" {
        # "Argument"
        # "Set Front Panel Open or Closed\n(Usage: \"UI: Front Panel State >> Open|Close\")"
        n132 = Unbundle By Name(w302) -> ("Core.Current VI Reference"=w301:refnum<vi>)
        n133 = case shown="\"Open\", Default" w300 {
          tunnel: w304 -> [w310 w323]
          tunnel: [w312 w324] -> w303
          tunnel: w301 -> [w311 w321]
          frame "Open", Default {
            n134 = property class="VI"(reference=w311, error in=w310) -> (reference out=w308:refnum<vi>, error out=w309:errorcluster, "Front Panel.Open"=w307:bool)
            n135 = case shown="False" w307 {
              tunnel: [w315 w318] -> w312
              tunnel: w309 -> [w314 w318]
              tunnel: w308 -> [w313 _]
              frame False {
                n136 = invoke class="VI" method="FP.Open"(reference=w313, error in=w314, "Activate"=TRUE, "State"=T5."Standard") -> (error out=w315:errorcluster)  [unwired: 1 in, 4 out]
              }
              frame True {
              }
            }
          }
          frame "Close" {
            n137 = property class="VI"(reference=w321, error in=w323) -> (reference out=w320:refnum<vi>, error out=w322:errorcluster, "Front Panel.Open"=w319:bool)
            n138 = case shown="True" w319 {
              tunnel: [w325 w328] -> w324
              tunnel: w322 -> [w325 w327]
              tunnel: w320 -> [_ w326]
              frame False {
              }
              frame True {
                n139 = invoke class="VI" method="FP.Close"(reference=w326, error in=w327) -> (error out=w328:errorcluster)  [unwired: 1 in, 2 out]
              }
            }
          }
        }
        n140 = call <vilib>:"Add State(s) to Queue__jki_lib_state_machine.vi"("State(s) in (\"\")"=w306) -> ("States Out"=w305:string)  [unwired: 14 in]
      }
      frame "---------- Macro ----------" {
        # "Do not put any code in this frame.\n(It is a separator no-op. You can make a copy of this frame to create a new Macro frame)"
        n141 = call <vilib>:"Add State(s) to Queue__jki_lib_state_machine.vi"("State(s) in (\"\")"=w332) -> ("States Out"=w331:string)  [unwired: 14 in]
      }
      frame "Macro: Initialize" {
        (unwired) "Data: Initialize\nInitialize Core Data\nUI: Initialize\nUI: Get Device Name\nUI: Update Device List\nUI: Start SuperGUI\nUI: Front Panel State >> Open\naction: update labels>>av1\naction:get status cmd\naction:send_cmd>>av1\naction:update status>>av1\naction:set to current values>>old"  # Data: Initialize Initialize Core Data UI: Initialize UI: Get Device Name UI: Update Device List UI: Start SuperGUI UI: Front Panel State >> Open action: update labels>>av1 action:get status cmd action:send_cmd>>av1 action:update status>>av1 action:set to current values>>old
        w333 = "Data: Initialize\nInitialize Core Data\nUI: Initialize\nUI: Get Device Name\nUI: Update Device List\nUI: Start SuperGUI\nUI: Front Panel State >> Open\naction: update labels>>av1"  # Data: Initialize Initialize Core Data UI: Initialize UI: Get Device Name UI: Update Device List UI: Start SuperGUI UI: Front Panel State >> Open action: update labels>>av1
        # "Initialization Macro\n(This is called once, when the VI starts)"
        n142 = call <vilib>:"Add State(s) to Queue__jki_lib_state_machine.vi"("State(s) in Front (\"\")"=w333, "State(s) in (\"\")"=w337) -> ("States Out"=w336:string)  [unwired: 13 in]
      }
      frame "Macro: Exit" {
        # "Exit Macro\n(This is called once, when the VI exits)"
        n143 = Unbundle By Name(w344) -> ("Core.Close Panel on Exit?"=w343:bool)
        n144 = Select(t="UI: Front Panel State >> Close", s=w343, f="") -> (s? t:f=w340:string)
        n145 = call <vilib>:"Add State(s) to Queue__jki_lib_state_machine.vi"("State(s) in (\"\")"=w340, "State(s) at Back (\"\")"="Data: Cleanup\nExit") -> ("States Out"=w338:string)  [unwired: 13 in]
        n146 = call <vilib>:"Add State(s) to Queue__jki_lib_state_machine.vi"("State(s) in Front (\"\")"=w338, "State(s) in (\"\")"=w347) -> ("States Out"=w346:string)  [unwired: 13 in]
      }
      frame "---------- New Category ----------" {
        # "Template Separator\n(You can make a copy of, or modify, this frame)"
        n147 = call <vilib>:"Add State(s) to Queue__jki_lib_state_machine.vi"("State(s) in (\"\")"=w351) -> ("States Out"=w350:string)  [unwired: 14 in]
      }
      frame "action:send_cmd" {
        # "Your code here.\n(You can make a copy of, or modify, this frame)"
        n148 = case shown="\"av1\"" w357 {
          tunnel: [_ "Avocent IP::1"] -> w363
          tunnel: [errorcluster {"status"=TRUE, "code"=0, "source"="Error:\nno avocent selected"} ("error out") w369] -> w355
          tunnel: w356 -> [_ w369]
          tunnel: ["" w368] -> w353
          tunnel: w354 -> [_ w368]
          frame Default {
          }
          frame "av1" {
          }
        }
        n149 = Unbundle By Name(w359) -> ("HTTP Command"=w361:string)
        n150 = call "Avocent_send_cmd.vi"("error in"=w355, "timeout ms"="timeout::1", "Avocent IP (in)"=w363, "HTTP command"=w361) -> ("error out"=w362:errorcluster, "Replay"=w360:string)  [unwired: 5 in, 1 out]
        n151 = Bundle By Name(cluster=w359, "Power Status"=w360) -> (w358:T6)
        n152 = call <vilib>:"Add State(s) to Queue__jki_lib_state_machine.vi"("State(s) in (\"\")"=w353) -> ("States Out"=w364:string)  [unwired: 14 in]
      }
      frame "Action:build_command_OFF" {
        # "Your code here.\n(You can make a copy of, or modify, this frame)"
        n153 = case shown="Default" w376 {
          tunnel: [_ "Set switches"] -> w371
          tunnel: ["" w384] -> w372
          tunnel: w375 -> [_ w384]
          tunnel: w374 -> [_ w383]
          tunnel: [errorcluster {"status"=TRUE, "code"=0, "source"="Error:\nno avocent selected"} ("error out") w383] -> w373
          frame Default {
          }
          frame "av1" {
          }
        }
        n154 = call "Avocent_build_command_OFF.vi"("Set switches"=w371) -> ("HTTP command"=w370:string)  [unwired: 10 in]
        n155 = Bundle By Name(cluster=w379, "Set Switch Status"=w371) -> (w378:T6)
        n156 = Bundle By Name(cluster=w378, "HTTP Command"=w370) -> (w377:T6)
        n157 = call <vilib>:"Add State(s) to Queue__jki_lib_state_machine.vi"("State(s) in (\"\")"=w372) -> ("States Out"=w380:string)  [unwired: 14 in]
      }
      frame "Action:build_command_ON" {
        # "Your code here.\n(You can make a copy of, or modify, this frame)"
        n158 = Unbundle By Name(w388) -> ("Set Switch Status"=w386:bool[])
        n159 = call "Avocent_build_command_ON.vi"("Set switches"=w386) -> ("HTTP command"=w387:string)  [unwired: 10 in]
        n160 = Bundle By Name(cluster=w388, "HTTP Command"=w387) -> (w389:T6)
        n161 = call <vilib>:"Add State(s) to Queue__jki_lib_state_machine.vi"("State(s) in (\"\")"=w392) -> ("States Out"=w391:string)  [unwired: 14 in]
      }
      frame "Action:build_command_toggle" {
        # "Your code here.\n(You can make a copy of, or modify, this frame)"
        n162 = case shown="Default" w399 {
          tunnel: [_ w409] -> w393
          tunnel: w401 -> [_ w408]
          tunnel: [errorcluster {"status"=TRUE, "code"=0, "source"="Error:\nno avocent selected"} ("error out") w407] -> w400
          tunnel: w397 -> [_ w406]
          tunnel: ["" w406] -> w396
          frame Default {
          }
          frame "av1" {
            n163 = property on="Set switches" class="Arr (strict)"(error in=w408) -> (error out=w407:errorcluster, "Value"=w409:bool[])  [unwired: 1 in, 1 out]
          }
        }
        n164 = Unbundle By Name(w398) -> ("Toggle On/Off"=w394:bool)
        n165 = call "Avocent_build_command_toggle.vi"("Set switches"=w393, "Toggle On/Off"=w394) -> ("HTTP Command"=w395:string)  [unwired: 9 in]
        n166 = Bundle By Name(cluster=w398, "HTTP Command"=w395) -> (w402:T6)
        n167 = call <vilib>:"Add State(s) to Queue__jki_lib_state_machine.vi"("State(s) in (\"\")"=w396) -> ("States Out"=w403:string)  [unwired: 14 in]
      }
      frame "action:update status" {
        # "Your code here.\n(You can make a copy of, or modify, this frame)"
        n168 = Unbundle By Name(w417) -> ("Power Status"=w410:string)
        n169 = call "Avocent_power_status.vi"("Power Status (raw string)"=w410) -> ("Power status (boolean)"=w411:bool[])  [unwired: 10 in]
        n170 = case shown="\"av1\"" w416 {
          tunnel: w411 -> [_ w423]
          tunnel: w415 -> [_ w422]
          tunnel: [errorcluster {"status"=TRUE, "code"=0, "source"="Error:\nno avocent selected"} ("error out") w422] -> w414
          tunnel: w413 -> [_ w421]
          tunnel: ["" w421] -> w412
          frame Default {
          }
          frame "av1" {
            "Power indicator" <- w423
          }
        }
        n171 = call <vilib>:"Add State(s) to Queue__jki_lib_state_machine.vi"("State(s) in (\"\")"=w412) -> ("States Out"=w418:string)  [unwired: 14 in]
      }
      frame "action:get status cmd" {
        # "Your code here.\n(You can make a copy of, or modify, this frame)"
        n172 = Bundle By Name(cluster=w426, "HTTP Command"="/control.cgi" ("Command")) -> (w425:T6)
        n173 = call <vilib>:"Add State(s) to Queue__jki_lib_state_machine.vi"("State(s) in (\"\")"=w429) -> ("States Out"=w428:string)  [unwired: 14 in]
      }
      frame "action:set to current values" {
        # "Your code here.\n(You can make a copy of, or modify, this frame)"
        n174 = case shown="\"old\"" w430 {
          tunnel: w432 -> [w453 w455]
          tunnel: [w453 w454] -> w431
          frame Default {
            n175 = local read "port: A::1"() -> (w437:bool)
            n176 = local read "port: B::1"() -> (w438:bool)
            n177 = local read "port: C::1"() -> (w439:bool)
            n178 = local read "port: D::1"() -> (w440:bool)
            n179 = local read "port: E::1"() -> (w441:bool)
            n180 = local read "port: F::1"() -> (w442:bool)
            n181 = local read "port: G::1"() -> (w443:bool)
            n182 = local read "port: H::1"() -> (w444:bool)
            n183 = local read "port: I::1"() -> (w445:bool)
            n184 = local read "port: J::1"() -> (w446:bool)
            n185 = local read "port: K::1"() -> (w447:bool)
            n186 = local read "port: L::1"() -> (w448:bool)
            n187 = local read "port: M::1"() -> (w449:bool)
            n188 = local read "port: N::1"() -> (w450:bool)
            n189 = local read "port: O::1"() -> (w451:bool)
            n190 = local read "port: P::1"() -> (w452:bool)
            n191 = Build Array(w437, w438, w439, w440, w441, w442, w443, w444, w445, w446, w447, w448, w449, w450, w451, w452) -> (w436:bool[])
            n192 = local write "Set switches"(w436) -> ()
          }
          frame "old" {
            n193 = property on="Power indicator" class="Arr (strict)"(error in=w455) -> (error out=w457:errorcluster, "Value"=w456:bool[])  [unwired: 1 in, 1 out]
            n194 = property on="Set switches" class="Arr (strict)"(error in=w457, "Val(Sgnl)"=w456) -> (error out=w454:errorcluster)  [unwired: 1 in, 1 out]
          }
        }
        n195 = call <vilib>:"Add State(s) to Queue__jki_lib_state_machine.vi"("State(s) in (\"\")"=w435) -> ("States Out"=w434:string)  [unwired: 14 in]
      }
      frame "action: set to all on/off" {
        # "Your code here.\n(You can make a copy of, or modify, this frame)"
        n196 = Unbundle By Name(w459) -> ("Set all On/Off"=w461:bool)
        n197 = Initialize Array(w461, 16 ("dimension size")) -> (w458:bool[])
        n198 = case shown="Default" w464 {
          tunnel: w466 -> [_ w472]
          tunnel: [errorcluster {"status"=TRUE, "code"=0, "source"="Error:\nno avocent selected"} ("error out") w471] -> w465
          tunnel: w463 -> [_ w473]
          tunnel: ["" w473] -> w462
          tunnel: w458 -> [_ w470]
          frame Default {
          }
          frame "av1" {
            n199 = property on="Set switches" class="Arr (strict)"(error in=w472, "Val(Sgnl)"=w470) -> (error out=w471:errorcluster)  [unwired: 1 in, 1 out]
          }
        }
        n200 = call <vilib>:"Add State(s) to Queue__jki_lib_state_machine.vi"("State(s) in (\"\")"=w462) -> ("States Out"=w467:string)  [unwired: 14 in]
      }
      frame "action: update labels" {
        n201 = call "get software root directory.vi"() -> ("Application Directory"=w485:path)  [unwired: 11 in]
        n202 = Strip Path(path=w485) -> (stripped path=w484:path)  [unwired: 1 out]
        n203 = Build Path(base path=w484, name or relative path="user data\\Avocent_PSU_Labels.txt") -> (appended path=w483:path)
        n204 = property on="GUIdevice 1" class="Str"(error in=w476) -> (error out=w475:errorcluster, "Value"=w474:string)  [unwired: 1 in, 1 out]
        n205 = call <vilib>:"Open Config Data.vi"("error in (no error)"=w475, "create file if necessary (T)"=FALSE, "configuration file path"=w483) -> ("error out"=w481:errorcluster, "refnum"=w482:T9)  [unwired: 6 in, 1 out]
        n206 = for {
          N: 16 -> [_]
          tunnel: w482 -> [w501]
          tunnel: w481 -> [w500]
          tunnel: [w499] -> w480
          tunnel: [w498] -> w479 mode=indexing
          tunnel: w474 -> [w491]
          i -> [w493]
          n207 = Add(x=w493, y=1) -> (x+y=w494:i32)
          n208 = Number To Decimal String(number=w494) -> (decimal integer string=w496:string)  [unwired: 1 in]
          n209 = Concatenate Strings("Label " ("key"), w496) -> (w495:string)
          n210 = call-poly <vilib>:"Read Key.vi"("section"=w491, "error in (no error)"=w500, "default value"="", "key"=w495, "refnum"=w501) -> ("error out"=w499:errorcluster, "value"=w498:string)  [unwired: 3 in, 2 out]
        }
        n211 = case shown="Default" w477 {
          tunnel: w479 -> [w490 _]
          frame "av1" {
            "Avocent Labels Av1" <- w490
          }
          frame Default {
          }
        }
      }
    }
  }
